vi "Subvi photoncounter.vi"(5 "DI channel":refnum<k21>="Connector0/DIO1", 12 "Photoncounter input selector":u8) -> (1 "PMT mon":bool, 2 "PMT edge change mon":bool, 3 "Gated pixelclock change mon":bool, 6 "Count":u8)   [LabVIEW 2017]
uses:
  <vilib>/rvi/eio/common/nirviEmuTemplateMethod_errors.vi
  GV PMT sim.vi
  GV gated pixelclock change.vi
  <vilib>/eio/EIONode/EIONode.xnode
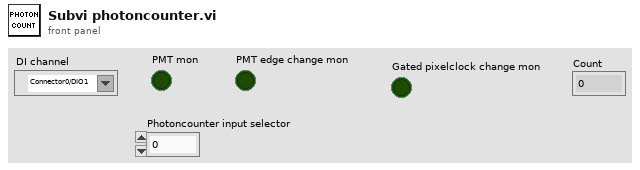
[diagram p1: front panel]
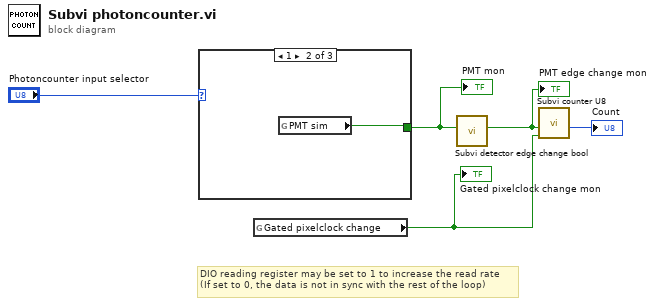
[diagram p0: block diagram]
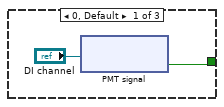
[diagram p2: hidden frame]
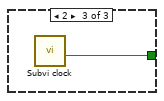
[diagram p3: hidden frame]
diagram:
  # "DIO reading register may be set to 1 to increase the read rate\n(If set to 0, the data is not in sync with the rest of the loop)"
  n1 = case shown="1" "Photoncounter input selector" {
    tunnel: [w6 w8 w9] -> w2
    frame 0, Default {
      n2 = xnode "PMT signal"("FPGA I/O In"="DI channel") -> ("I/O Item"=w6:bool)  [unwired: 1 out]
    }
    frame 1 {
      n3 = global read "GV PMT sim.vi" "PMT sim"() -> (w8:bool)
    }
    frame 2 {
      n4 = call "Subvi clock.vi"() -> ("Output"=w9:bool)  [unwired: 11 in]
    }
  }
  "PMT mon" <- w2
  n5 = global read "GV gated pixelclock change.vi" "Gated pixelclock change"() -> (w5:bool)
  "Gated pixelclock change mon" <- w5
  n6 = call "Subvi detector edge change bool.vi"("Input"=w2) -> ("Output"=w1:bool)  [unwired: 8 in]
  "PMT edge change mon" <- w1
  n7 = call "Subvi counter U8.vi"("Reset"=w5, "+1"=w1) -> ("Count"=→"Count":u8)  [unwired: 9 in]
